vi "FlatToRichhelloworld_HelloReply.vi"(5 "OutputClusterType":T1, 11 "InputCluster":T2) -> (3 "OutputCluster":T1)   [LabVIEW 2019, in "helloworld_server.lvlib"]
uses:
  helloworld_server.lvlib
  helloworld_HelloReply_Flat.ctl
  helloworld_HelloReply.ctl
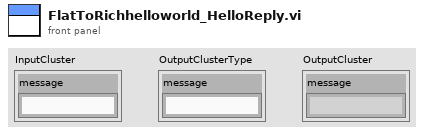
[diagram p1: front panel]
types:
  T1 = typedef "helloworld_server.lvlib/helloworld_HelloReply.ctl" = cluster{"message":string}
  T2 = typedef "helloworld_server.lvlib/helloworld_HelloReply_Flat.ctl" = cluster{"message":string}
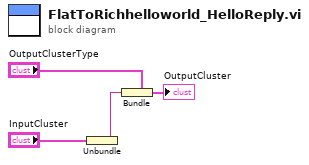
[diagram p0: block diagram]
diagram:
  n1 = Unbundle "Unbundle"("InputCluster") -> ("message"=w1:string)
  n2 = Bundle "Bundle"(cluster="OutputClusterType", "message"=w1) -> (→"OutputCluster":T1)
